vi "GageAvgSpec_test_och.vi"() -> ()   [LabVIEW 2016]
uses:
  <vilib>/express/express analysis/Spectral/XNode/ExpressSpectralMeasurementsBlockNode.xnode
  <vilib>/express/express analysis/Spectral/Block/exnSpectralBlock spectral measurements power poly.vi
  <vilib>/express/express analysis/Spectral/Block/exnSpectralBlock spectral measurements power WFM.vi
  <vilib>/Utility/file.llb/Write To Spreadsheet File (DBL).vi
panel:
  in  "Start 4":i32
  in  "Points 4":u32=4096
  in  "Averages 5":u32=1 min=1 step=1
  out "Spec(ch3) 4":cluster{"f0":dbl, "df":dbl, "magnitude":dbl[]}(graph)
  out "Spec(ch2) 4":cluster{"f0":dbl, "df":dbl, "magnitude":dbl[]}(graph)
  out "Spec(ch0) 4":cluster{"f0":dbl, "df":dbl, "magnitude":dbl[]}(graph)
  in  "데이터 저장 시작 3":bool
  out "100 세트 저장완료 3":bool
  out "System Count":i32
  out "Progress 3":string
  in  "stop 3":bool
  in  "Channels 2":T1(array[cluster])=[{"Coupling"=0, "Differential Input"=FALSE, "Direct-to-ADC"=FALSE, "Range"=2000, "Impedance"=50, "Filter"=0}] {"Impedance" min=50 max=1000000 step=999950; "Coupling" items=["DC", "AC"]}
  in  "Trigger":T2={"Slope"=0, "Level"=0, "Source"=0, "External Range"=2000, "External Coupling"=0, "External"=FALSE, "Disable"=FALSE, "External Impedance"=1} {"External Impedance" items=["50 Ohm", "HiZ"]; "External Coupling" items=["DC", "AC"]; "External Range" min=2000 max=10000 step=8000; "Slope" items=["Rising", "Falling"]; "Level" min=-100 max=100; "Source" min=0 max=64 step=1}
  in  "Acquisition 2":T3={"Sample Rate"=50000000.0, "Mode"=2, "Depth"=8192.0, "Segment Size"=8192.0, "Trigger Timeout"=1000000.0, "Trigger Holdoff"=0.0, "Trigger Delay"=0.0, "Clock mode"=enum."Internal"} {"Segment Size" min=256.0 step=128.0; "Trigger Holdoff" min=0.0 step=128.0; "Trigger Delay" min=0.0 step=128.0; "Depth" min=256.0 step=128.0; "Mode" items=["Single", "Dual", "Quad", "Octal"]}
  in  "Averages":u32=1 min=1 step=1
  in  "Averaging Method":bool
  out "Sample Bits 2":i32
  out "Board Count 2":i32
  out "Channel Count 2":i32
  out "Trigger Count 2":i32
  out "System Name 2":string
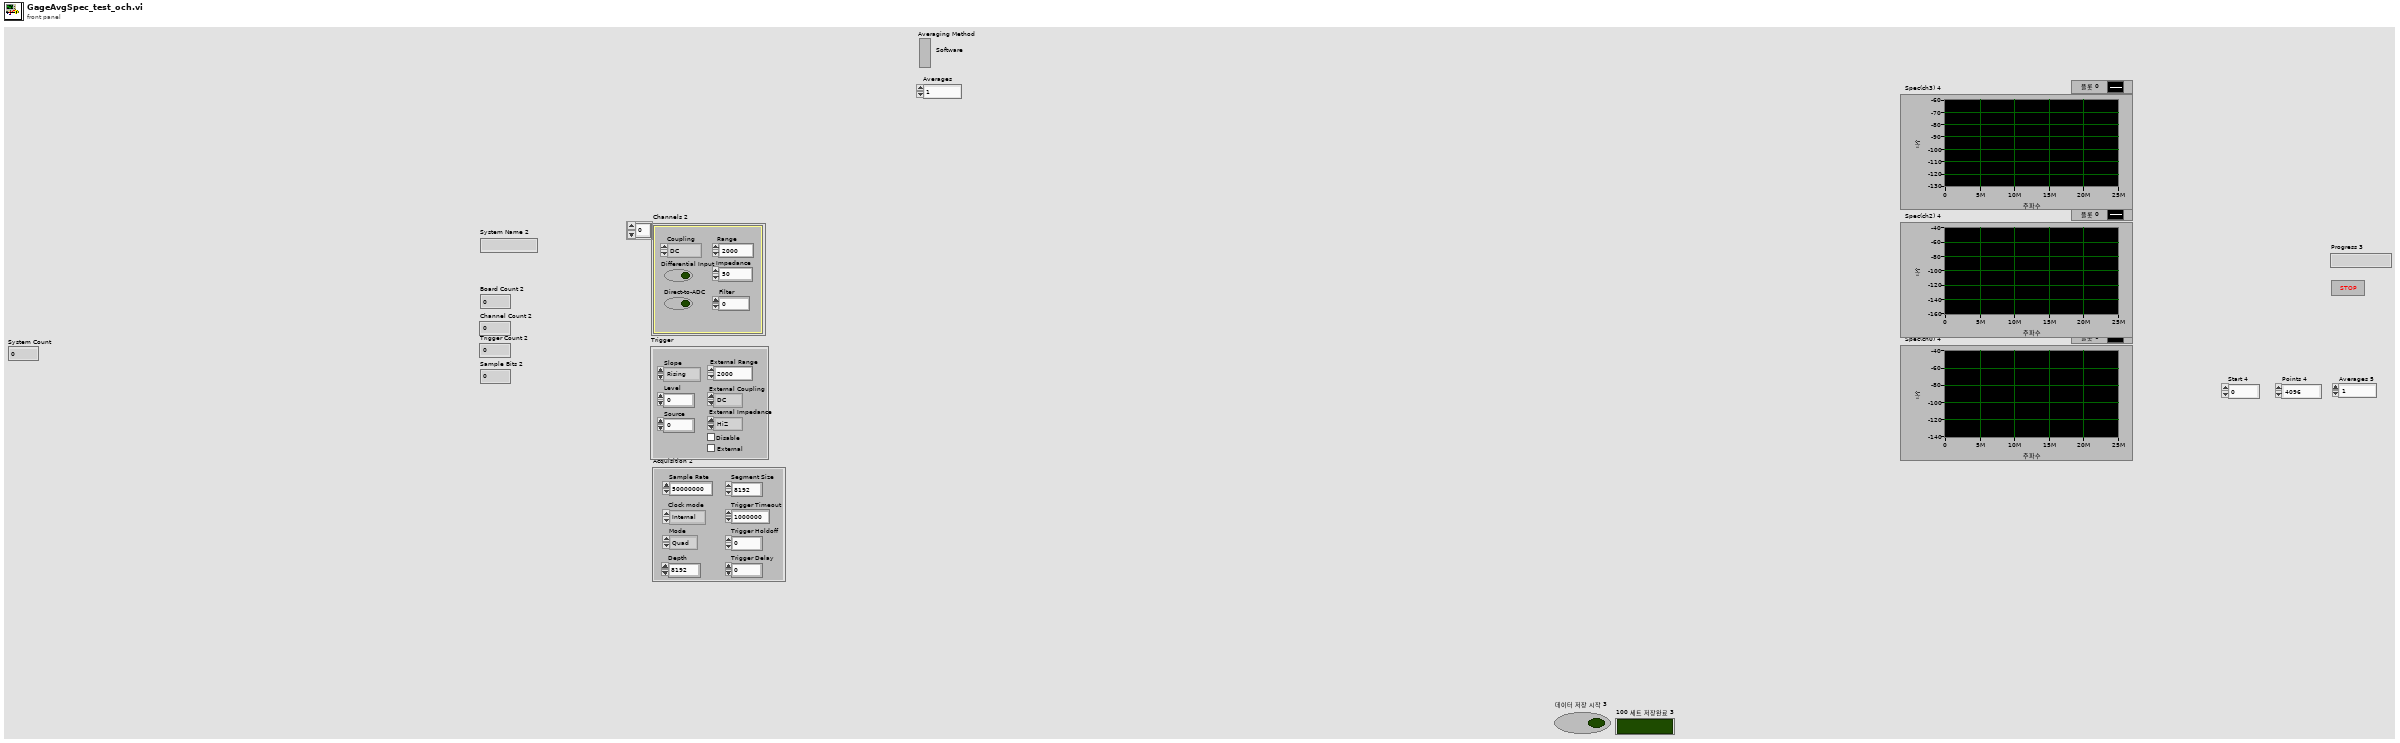
[diagram p1: front panel]
types:
  T1 = cluster{"Coupling":u16, "Differential Input":bool, "Direct-to-ADC":bool, "Range":u32, "Impedance":u32, "Filter":i32}[]
  T2 = cluster{"Slope":u16, "Level":i32, "Source":i32, "External Range":u32, "External Coupling":u16, "External":bool, "Disable":bool, "External Impedance":u16}
  T3 = cluster{"Sample Rate":dbl, "Mode":u16, "Depth":dbl, "Segment Size":dbl, "Trigger Timeout":dbl, "Trigger Holdoff":dbl, "Trigger Delay":dbl, "Clock mode":enum16{"Internal", "External", "Reference"}}
  T4 = cluster{"averaging mode":u16, "weighting mode":u16, "number of averages":u32}
  T5 = cluster{"dB On (F)":bool, "unwrap phase (F)":bool, "convert to degree (F)":bool}
  T6 = cluster{"Handle":u32, "Sample size":u32, "Resolution":i32, "Offset":i32, "Channels":u32, "Boards":u32}
  T7 = cluster{string, "Differential Input":bool, "Direct-to-ADC":bool, "Range":u32, "Impedance":u32, i32, "Filter":i32}
  T8 = cluster{"RingText.Text":string, "Level":i32, "Source":i32, "External Range":u32, "RingText.Text":string, "External":bool, "Disable":bool, "RingText.Text":string}
  T9 = cluster{"RingText.Text":string, "Level":i32, "Source":i32, "External Range":u32, "RingText.Text":string, "External":bool, "Disable":bool, "RingText.Text":string}[]
  T10 = cluster{"Handle":u32, "Sample Size":u32, "Resolution":i32, "Offset":i32, "Channels":u32, "Boards":u32}
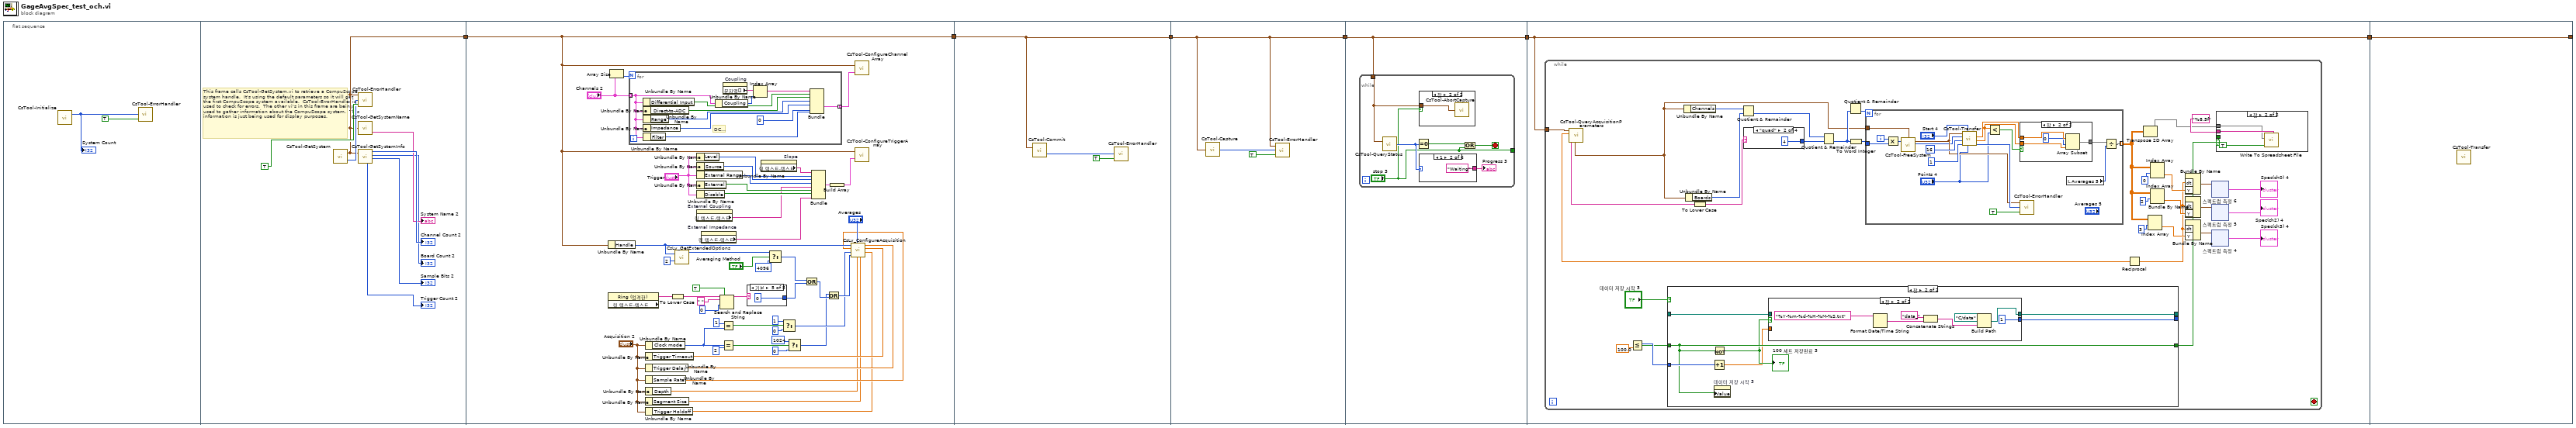
[diagram p0: block diagram]
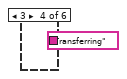
[diagram p9: hidden frame]
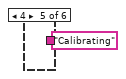
[diagram p10: hidden frame]
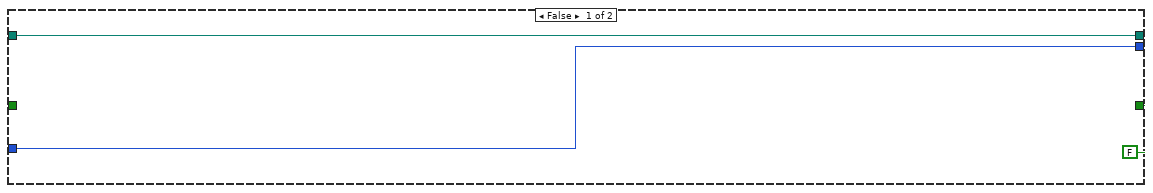
[diagram p12: hidden frame]
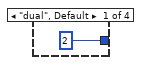
[diagram p15: hidden frame]
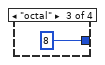
[diagram p16: hidden frame]
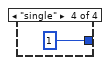
[diagram p17: hidden frame]
diagram:
  n1 = flat-sequence {
    tunnel: [w9] -> w6
    tunnel: w6 -> [w64]
    tunnel: [w64] -> w5
    tunnel: w5 -> [w83]
    tunnel: [w83] -> w4
    tunnel: w4 -> [w85]
    tunnel: [w85] -> w3
    tunnel: w3 -> [w87]
    tunnel: [w87] -> w2
    tunnel: w2 -> [w101]
    tunnel: [w101] -> w1
    tunnel: w1 -> [w208]
    tunnel: [w208] -> _
    frame #0 {
      n2 = call <userlib>:"CsTool-Initialize.vi"() -> ("Number Of Systems"=w8:i32)  [unwired: 1 out]
      "System Count" <- w8
      n3 = call <userlib>:"CsTool-ErrorHandler.vi"("StopOnError (true)"=TRUE, "Error Code"=w8) -> ()  [unwired: 1 in, 1 out]
    }
    frame #1 {
      # "This frame calls CsTool-GetSystem.vi to retrieve a CompuScope system handle.  It's using the default parameters so it will get the first CompuScope system available.  CsTool-ErrorHandler is used to check for errors.  The other vi's in this frame are being used to gather information about the CompuScope system.  This information is just being used for display purposes."
      n4 = call <userlib>:"CsTool-GetSystem.vi"() -> ("Error Code"=w10:i32, "Handle Cluster"=w9:T6)  [unwired: 4 in]
      n5 = call <userlib>:"CsTool-ErrorHandler.vi"("StopOnError (true)"=TRUE, "Error Code"=w10, "Handle Cluster"=w9) -> ()  [unwired: 1 out]
      n6 = call <userlib>:"CsTool-GetSystemName.vi"("Handle Cluster"=w9) -> ("System Name"=→"System Name 2":string)  [unwired: 1 out]
      n7 = call <userlib>:"CsTool-GetSystemInfo.vi"("Handle Cluster"=w9) -> ("Number Of Triggers"=→"Trigger Count 2":u32, "Number Of Channels"=→"Channel Count 2":u32, "Number Of Boards"=→"Board Count 2":u32, "Sample Bits"=→"Sample Bits 2":u32)  [unwired: 3 out]
    }
    frame #2 {
      n8 = Unbundle By Name(w64) -> ("Handle"=w58:u32)
      n9 = property on="프로퍼티 노드" class="Ring (엄격한)"() -> ("링 텍스트.텍스트"=w61:string)  [unwired: 2 in, 2 out]
      n10 = Array Size(array="Channels 2") -> (size(s)=w18:i32)
      n11 = for {
        N: w18 -> [_]
        tunnel: "Channels 2" -> [w68] mode=indexing
        tunnel: [w72] -> w17 mode=indexing
        # "DC Offset"
        n12 = Unbundle By Name(w68) -> ("Differential Input"=w75:bool)
        n13 = Unbundle By Name(w68) -> ("Direct-to-ADC"=w74:bool)
        n14 = Unbundle By Name(w68) -> ("Range"=w65:u32)
        n15 = Unbundle By Name(w68) -> ("Impedance"=w73:u32)
        n16 = Unbundle By Name(w68) -> ("Filter"=w67:i32)
        n17 = Unbundle By Name(w68) -> ("Coupling"=w70:u16)
        n18 = property on="Coupling" class="Ring (엄격한)"() -> ("문자열[]"=w71:string[])  [unwired: 2 in, 2 out]
        n19 = Index Array(array=w71, index=w70) -> (element=w69:string)
        n20 = Bundle(w69, "Differential Input"=w75, "Direct-to-ADC"=w74, "Range"=w65, "Impedance"=w73, 0, "Filter"=w67) -> (w72:T7)  [unwired: 1 in]
      }
      n21 = Unbundle By Name("Acquisition 2") -> ("Trigger Timeout"=w49:dbl)
      n22 = Unbundle By Name("Acquisition 2") -> ("Segment Size"=w33:dbl)
      n23 = Unbundle By Name("Acquisition 2") -> ("Trigger Holdoff"=w32:dbl)
      n24 = Unbundle By Name("Acquisition 2") -> ("Clock mode"=w37:enum16{"Internal", "External", "Reference"})
      n25 = Unbundle By Name("Acquisition 2") -> ("Trigger Delay"=w48:dbl)
      n26 = Unbundle By Name("Acquisition 2") -> ("Sample Rate"=w47:dbl)
      n27 = Unbundle By Name("Acquisition 2") -> ("Depth"=w34:dbl)
      n28 = To Lower Case(string=w61) -> ()  [unwired: 1 out]
      n29 = call <userlib>:"CsLv_GetExtendedOptions.vi"("Handle"=w58, "Option"=2) -> ("User Mode"=w56:u32)  [unwired: 2 out]
      n30 = property on="External Coupling" class="Ring (엄격한)"() -> ("링 텍스트.텍스트"=w22:string)  [unwired: 2 in, 2 out]
      n31 = Unbundle By Name("Trigger") -> ("Level"=w30:i32)
      n32 = Unbundle By Name("Trigger") -> ("Source"=w27:i32)
      n33 = Unbundle By Name("Trigger") -> ("External Range"=w29:u32)
      n34 = Unbundle By Name("Trigger") -> ("External"=w26:bool)
      n35 = Unbundle By Name("Trigger") -> ("Disable"=w25:bool)
      n36 = property on="External Impedance" class="Ring (엄격한)"() -> ("링 텍스트.텍스트"=w21:string)  [unwired: 2 in, 2 out]
      n37 = Search and Replace String(replace all?=TRUE, input string=w61, search string=" ", offset=0) -> (result string=w60:string)  [unwired: 4 in, 3 out]
      n38 = Equal?(x=1, y=w37) -> (x = y?=w41:bool)
      n39 = Equal?(x=w37, y=2) -> (x = y?=w39:bool)
      n40 = case shown="기본" w60 {
        tunnel: [1 2 4 8 0] -> w52
        frame "single" {
        }
        frame "dual" {
        }
        frame "quad" {
        }
        frame "octal" {
        }
        frame Default {
        }
      }
      n41 = property on="Slope" class="Ring (엄격한)"() -> ("링 텍스트.텍스트"=w23:string)  [unwired: 2 in, 2 out]
      n42 = Select(t=w56, s="Averaging Method", f=4096) -> (s? t:f=w53:u32)
      n43 = Select(t=u32 1, s=w41, f=u32 0) -> (s? t:f=w36:u32)
      n44 = Select(t=1024, s=w39, f=0) -> (s? t:f=w35:i32)
      n45 = Or(x=w53, y=w52) -> (x .or. y?=w54:u32)
      n46 = Bundle("RingText.Text"=w23, "Level"=w30, "Source"=w27, "External Range"=w29, "RingText.Text"=w22, "External"=w26, "Disable"=w25, "RingText.Text"=w21) -> (w28:T8)  [unwired: 1 in]
      n47 = Or(x=w35, y=w54) -> (x .or. y?=w51:u32)
      n48 = Build Array(w28) -> (w20:T9)
      n49 = call <userlib>:"CsLv_ConfigureAcquisition.vi"("Trigger Holdoff (0)"=w32, "Trigger Timeout (10000000)"=w49, "Trigger Delay (0)"=w48, "Segment Size (8192)"=w33, "Depth (8192)"=w34, "Segment Count (1)"="Averages", "Mode (2)"=w51, "External Clock (0)"=w36, "Sample Rate (100000000)"=w47, "Handle"=w58) -> ()  [unwired: 1 in, 1 out]
      n50 = call <userlib>:"CsTool-ConfigureChannelArray.vi"("Channels"=w17, "Handle Cluster"=w64) -> ()  [unwired: 1 out]
      n51 = call <userlib>:"CsTool-ConfigureTriggerArray.vi"("Triggers"=w20, "Handle Cluster"=w64) -> ()  [unwired: 1 out]
    }
    frame #3 {
      n52 = call <userlib>:"CsTool-Commit.vi"("Handle Cluster"=w83) -> ("Error Code"=w81:i32)  [unwired: 2 in, 1 out]
      n53 = call <userlib>:"CsTool-ErrorHandler.vi"("StopOnError (true)"=TRUE, "Error Code"=w81) -> ()  [unwired: 1 in, 1 out]
    }
    frame #4 {
      n54 = call <userlib>:"CsTool-Capture.vi"("Handle Cluster"=w85) -> ("Error Code"=w84:i32)
      n55 = call <userlib>:"CsTool-ErrorHandler.vi"("StopOnError (true)"=TRUE, "Error Code"=w84, "Handle Cluster"=w85) -> ()  [unwired: 1 out]
    }
    frame #5 {
      n56 = while {
        tunnel: ["stop 3"] -> _
        tunnel: w87 -> [w88]
        stop <- w90 stop-if-true
        n57 = call <userlib>:"CsTool-QueryStatus.vi"("Handle Cluster"=w88) -> ("Status"=w93:i32)
        n58 = Equal To 0?(x=w93) -> (x = 0?=w91:bool)
        n59 = case shown="참" "stop 3" {
          tunnel: w88 -> [_ w94]
          frame False {
          }
          frame True {
            n60 = call <userlib>:"CsTool-AbortCapture.vi"("Handle Cluster"=w94) -> ()  [unwired: 1 out]
          }
        }
        n61 = case shown="1" w93 {
          tunnel: ["Ready" "Waiting" "Triggered" "Transferring" "Calibrating" " "] -> w92
          frame 0 {
          }
          frame 1 {
          }
          frame 2 {
          }
          frame 3 {
          }
          frame 4 {
          }
          frame 5, Default {
          }
        }
        "Progress 3" <- w92
        n62 = Or(x=w91, y="stop 3") -> (x .or. y?=w90:bool)
      }
    }
    frame #6 {
      n63 = while {
        tunnel: w101 -> [w102]
        stop <- _ stop-if-true
        n64 = call <userlib>:"CsTool-QueryAcquisitionParameters.vi"("Handle Cluster"=w102) -> ("Output Handle Cluster"=w109:T10, "Mode"=w110:string, "Sample Rate"=w108:dbl)  [unwired: 8 out]
        n65 = Unbundle By Name(w109) -> ("Channels"=w128:u32)
        n66 = Unbundle By Name(w109) -> ("Boards"=w131:u32)
        n67 = To Lower Case(string=w110) -> (all lower case string=w132:string)
        n68 = Quotient & Remainder(x=w128, y=w131) -> (floor(x/y)=w130:u32)  [unwired: 1 out]
        n69 = case shown="\"quad\"" w132 {
          tunnel: [2 4 8 1] -> w129
          frame "dual", Default {
          }
          frame "quad" {
          }
          frame "octal" {
          }
          frame "single" {
          }
        }
        n70 = Quotient & Remainder(x=w130, y=w129) -> (floor(x/y)=w127:u32)  [unwired: 1 out]
        n71 = Quotient & Remainder(y=w127) -> (floor(x/y)=w126:u32)  [unwired: 1 in, 1 out]
        n72 = To Word Integer(number=w127) -> (16bit integer=w133:i16)
        n73 = for {
          N: w126 -> [_]
          tunnel: w109 -> [w192]
          tunnel: [w188] -> w111 mode=indexing
          tunnel: w133 -> [w193]
          i -> [w201]
          n74 = Multiply(x=w201, y=w193) -> (x*y=w191:i32)
          n75 = call <userlib>:"CsTool-Transfer.vi"("Length (4096)"="Points 4", "Start (0)"="Start 4", "Segment (1)"=1, "Mode (0)"=16, "Channel (0)"=w191, "Handle Cluster"=w192) -> ("Error Code"=w196:i32, "Actual Length"=w199:dbl, "Data in Volts"=w189:dbl[])  [unwired: 1 out]
          n76 = Less?(x=w199, y="Points 4") -> (x < y?=w202:bool)
          n77 = case shown="참" w202 {
            tunnel: w189 -> [w203 w207]
            tunnel: w199 -> [_ w205]
            tunnel: [w203 w204] -> w190
            frame False {
            }
            frame True {
              n78 = Array Subset(array=w207, index=0, length=w205) -> (w204:dbl[])
            }
          }
          n79 = call <userlib>:"CsTool-ErrorHandler.vi"("StopOnError (true)"=TRUE, "Error Code"=w196, "Handle Cluster"=w192) -> ()  [unwired: 1 out]
          n80 = local read "Averages 5"() -> (w194:u32)
          n81 = Divide(x=w190, y=w194) -> (x/y=w188:dbl[])
        }
        n82 = Reciprocal() -> ()  [unwired: 1 in, 1 out]
        n83 = Transpose 2D Array(2D array=w111) -> (transposed array=w115:dbl[][])
        n84 = Index Array(array=w111, index (row)=3 ("인덱스 (행)")) -> (element=w119:dbl[])  [unwired: 1 in]
        n85 = Index Array(array=w111, index (row)=0 ("인덱스 (행)")) -> (element=w123:dbl[])  [unwired: 1 in]
        n86 = Index Array(array=w111, index (row)=2 ("인덱스 (행)")) -> (element=w121:dbl[])  [unwired: 1 in]
        n87 = Bundle By Name("dt"=w108, "Y"=w123) -> (w124:waveform(dbl))  [unwired: 1 in]
        n88 = Bundle By Name("dt"=w108, "Y"=w121) -> (w122:waveform(dbl))  [unwired: 1 in]
        n89 = Bundle By Name("dt"=w108, "Y"=w119) -> (w120:waveform(dbl))  [unwired: 1 in]
        n90 = xnode "스펙트럼 측정 6"("신호"=w124) -> ("파워 스펙트럼"=→"Spec(ch0) 4":cluster{"f0":dbl, "df":dbl, "magnitude":dbl[]})  [unwired: 1 in, 1 out]
        n91 = xnode "스펙트럼 측정 5"("신호"=w122) -> ("파워 스펙트럼"=→"Spec(ch2) 4":cluster{"f0":dbl, "df":dbl, "magnitude":dbl[]})  [unwired: 1 in, 1 out]
        n92 = xnode "스펙트럼 측정 4"("신호"=w120) -> ("파워 스펙트럼"=→"Spec(ch3) 4":cluster{"f0":dbl, "df":dbl, "magnitude":dbl[]})  [unwired: 1 in, 1 out]
        n93 = Less Or Equal?(x=w107, y=100.0) -> (x <= y?=w106:bool)
        n94 = case shown="참" "데이터 저장 시작 3" {
          tunnel: [FALSE w142] -> w103
          tunnel: w106 -> [_ w142]
          tunnel: [w136 w139] -> _
          tunnel: [w136 w143] -> w107
          tunnel: [w134 w138] -> _
          tunnel: [w134 w137] -> _
          frame False {
          }
          frame True {
            n95 = Increment(x=w143) -> (x+1=w140:dbl)
            n96 = Not(x=w142) -> (.not. x?=w141:bool)
            "100 세트 저장완료 3" <- w141
            n97 = property on="데이터 저장 시작 3" class="Bool (엄격한)"("Value"=w142) -> ()  [unwired: 2 in, 2 out]
            n98 = case shown="참" w141 {
              tunnel: [w145 1] -> w139
              tunnel: w140 -> [w145 _]
              tunnel: [w144 _] -> w138
              tunnel: [w144 w146] -> w137
              frame False {
              }
              frame True {
                n99 = Format Date/Time String(time format string (%c)="%Y-%m-%d-%H-%M-%S.txt" ("시간 포맷 문자열 (%c)")) -> (date/time string=w148:string)  [unwired: 2 in]
                n100 = Concatenate Strings("data_", w148) -> (w147:string)
                n101 = Build Path(base path=path "C:/data", name or relative path=w147) -> (appended path=w146:path)
              }
            }
          }
        }
        n102 = case shown="참" {
          selector: _ -> [_ _]
          tunnel: w103 -> [_ _]
          tunnel: "%8.5f" ("format (%.3f)") -> [_ w154]
          tunnel: w115 -> [_ w153]
          frame False {
          }
          frame True {
            n103 = call-poly <vilib>:"Write To Spreadsheet File.vi"("format (%.3f)"=w154, "append to file? (new file:F)"=TRUE, "2D data"=w153) -> ()  [unwired: 5 in, 1 out]
          }
        }
      }
    }
    frame #7 {
      n104 = call <userlib>:"CsTool-Transfer.vi"() -> ()  [unwired: 6 in, 4 out]
    }
  }
  n105 = call <userlib>:"CsTool-FreeSystem.vi"() -> ()  [unwired: 1 in, 1 out]
